vi "Build Installer with API.vi"(8 "error in (no error)":errorcluster, 11 "PostBuildSupport in":refnum<class "PostBuildSupport.lvclass">) -> (0 "error out":errorcluster, 3 "PostBuildSupport out":refnum<class "PostBuildSupport.lvclass">)   [LabVIEW 2016, in "PostBuildSupport.lvclass"]
uses:
  PostBuildSupport.lvclass
  PostBuildSupport.lvclass/PostBuildSupport.ctl
  <vilib>/AppBuilder/IB_Classes/Destination/IB_Destination.lvclass
  <vilib>/AppBuilder/IB_Classes/Source/IB_Source.lvclass
  <vilib>/AppBuilder/IB_Classes/Dest_NI_NIPath/Dest_NI_NIPath.lvclass
  <vilib>/AppBuilder/AB_API/EXE/NI_AB_API_EXE.lvclass
  <vilib>/AppBuilder/IB_Classes/Installer/Installer.lvclass
panel:
  in  "Cancel Button":bool
  out "Progress Bar":u8(slide) caption="The build is complete. You can locate the build at\nC:\\user\\patrick\\git\\PPMS-Monitor-and-Control\\builds\\PPMS Monitor and Control\\Application." scale=0.0..100.0
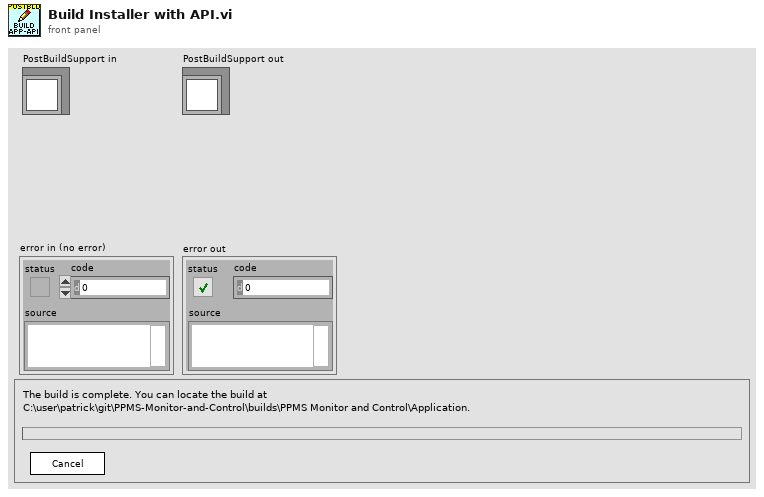
[diagram p1: front panel]
types:
  T1 = enum8{"Enabled", "Disabled", "Disabled and Grayed Out"}
  T2 = typedef "IB_Installer.ctl" = cluster{"Destination":refnum<class "IB_Destination.lvclass">[], "Source":refnum<class "IB_Source.lvclass">[], "buildObject":T3, "defaultDir":string, "platform":string, "author":string, "productName":string, "buildSpecName":string, "hide":bool, "requireLVDevSys":bool, "autoIncrement":bool, "includeError":bool, "readmeID":string, "buildLocation":path, "readmePath":path, "mediaSize":u16, "language":T4, "productVersion":T5, "preview":bool, "programmatic":bool, "progressBarEvents":T6, "userLog_Path":path, "shortcutAddresses":T8[], "EXE_Install Address":string, "EXE_Uninstall Address":string, "additional NIPaths":refnum<class "Dest_NI_NIPath.lvclass">[], "web service itemIDs":string[]}
  T3 = typedef "ItemRef.ctl" = u64
  T4 = typedef "CDK_sTypeDef_Languages.ctl" = u16
  T5 = typedef "CDK_sTypeDef_ProductVersion.ctl" = cluster{"Major":u8, "Minor":u8, "Update":u16}
  T6 = typedef "provcom_ProgressBar_Events.ctl" = cluster{"newJob":refnum<user-event>, "newItem":refnum<user-event>, "errorMsg":T7, "cancel":refnum<user-event>}
  T7 = typedef "mxLvBuildError.ctl" = refnum<user-event>
  T8 = typedef "CDK_sTypeDef_ShortcutAddress.ctl" = cluster{"file":string, "shortcut":string}
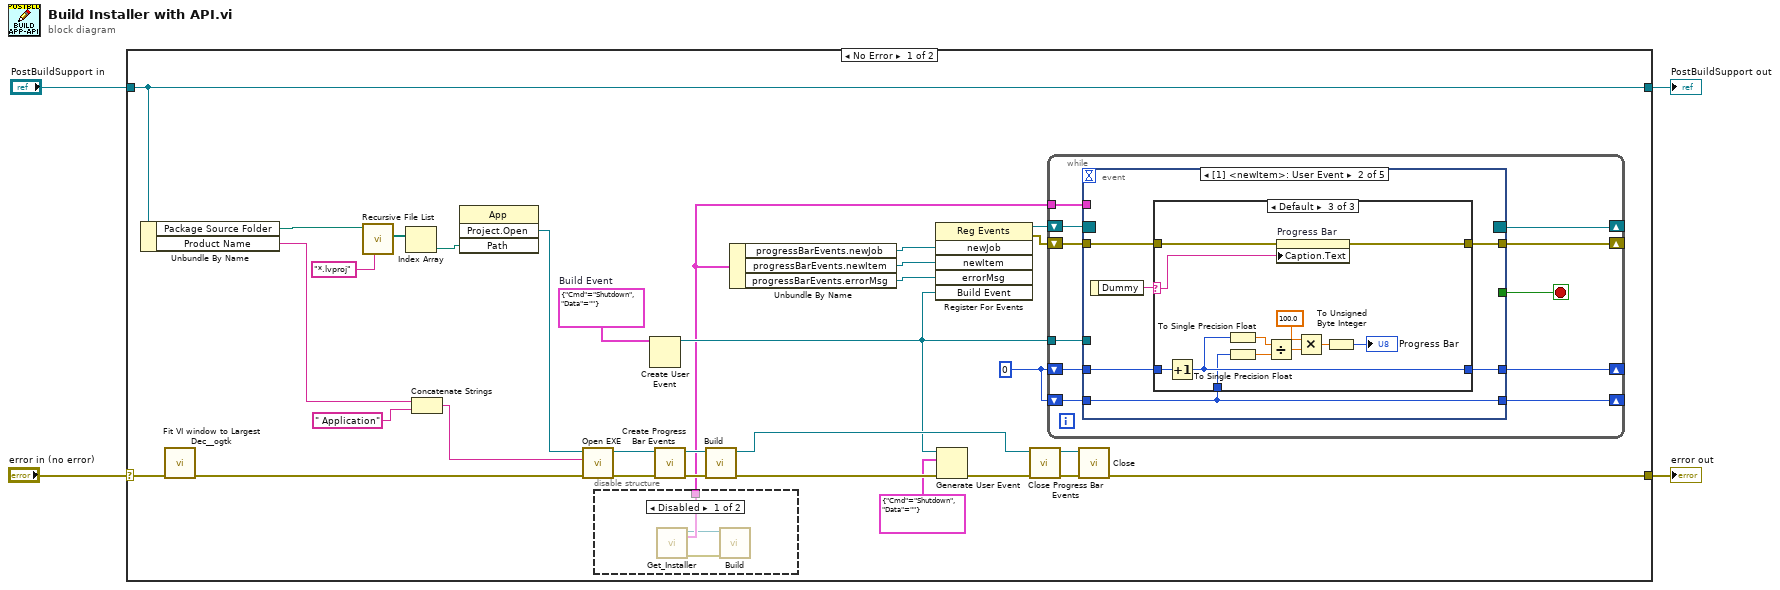
[diagram p0: block diagram]
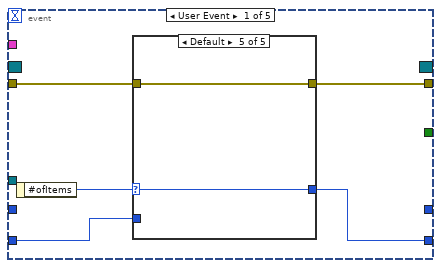
[diagram p3: hidden frame]
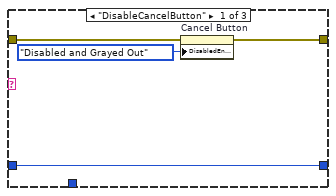
[diagram p8: hidden frame]
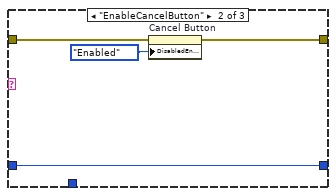
[diagram p9: hidden frame]
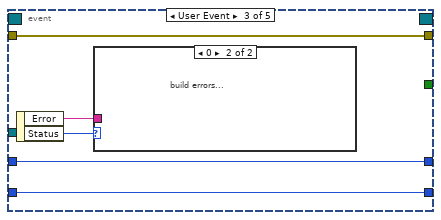
[diagram p10: hidden frame]
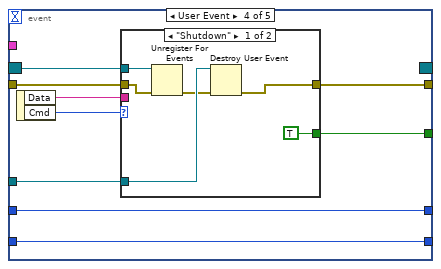
[diagram p12: hidden frame]
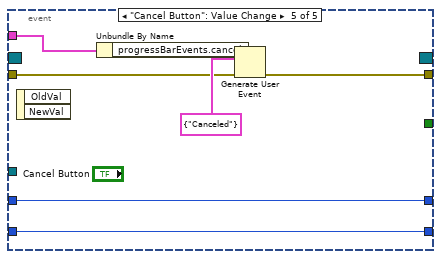
[diagram p14: hidden frame]
diagram:
  n1 = case shown="No Error" "error in (no error)" {
    selector: "error in (no error)" -> [w25 w120]
    tunnel: "PostBuildSupport in" -> [w34 w119]
    tunnel: [w32 w120] -> w2
    tunnel: [w34 w119] -> w1
    frame No Error {
      w13 = cluster{"Cmd":enum16{"Shutdown"}, "Data":string} {"Cmd"=enum."Shutdown", "Data"=""}  # Build Event
      w12 = 0 ("#ofItems")
      n2 = Unbundle By Name(w34) -> ("Package Source Folder"=w28:path, "Product Name"=w29:string)
      n3 = call <userlib>:"Fit VI window to Largest Dec__ogtk.vi"("error in (no error)"=w25) -> ("error out"=w24:errorcluster)  [unwired: 5 in, 1 out]
      n4 = call <vilib>:"Recursive File List.vi"("pattern"="*.lvproj", "Folder Path"=w28) -> ("All Files in Dir"=w35:path[])  [unwired: 5 in, 4 out]
      n5 = Index Array(array=w35) -> (element=w31:path)  [unwired: 1 in]
      n6 = Concatenate Strings(w29, " Application" ("Name of target (My Computer)")) -> (w27:string)
      n7 = invoke class="App" method="Project.Open"("Path"=w31) -> ("Project:Open"=w30:refnum<vi>)  [unwired: 3 in, 3 out]
      n8 = call <vilib>:"Open EXE.vi"("error in (no error)"=w24, "Build specification name"=w27, "Project Refnum"=w30) -> ("error out"=w7:errorcluster, "EXE out"=w5:refnum<class "NI_AB_API_EXE.lvclass">)  [unwired: 7 in]
      n9 = disable-structure shown="Disabled" {
        disable-tunnel: [w38 _] -> w6
        frame Disabled {
          n10 = call <vilib>:"Get_Installer.vi"() -> ("error out"=w37:errorcluster, "data"=w38:T2, "Installer out"=w36:refnum<class "Installer.lvclass">)  [unwired: 9 in]
          n11 = call-dynamic "Build.vi"("error in (no error)"=w37, "Class in"=w36) -> ()  [unwired: 6 in, 4 out]
        }
        frame Enabled {
        }
      }
      n12 = Create User Event(user event datatype=w13) -> (user event=w9:refnum<user-event>)  [unwired: 1 in, 1 out]
      n13 = call-dynamic "Create Progress Bar Events.vi"("error in (no error)"=w7, "NI_AB_API_Build in"=w5) -> ("error out"=w19:errorcluster, "NI_AB_API_Build out"=w23:refnum<class "NI_AB_API_EXE.lvclass">)  [unwired: 7 in, 1 out]
      n14 = call-dynamic "Build.vi"("error in (no error)"=w19, "EXE in"=w23) -> ("error out"=w11:errorcluster, "EXE out"=w22:refnum<class "NI_AB_API_EXE.lvclass">)  [unwired: 6 in, 2 out]
      n15 = Unbundle By Name(w6) -> ("progressBarEvents.newJob"=w18:refnum<user-event>, "progressBarEvents.newItem"=w17:refnum<user-event>, "progressBarEvents.errorMsg"=w16:T7)
      n16 = register-events(w18, w17, w16, w9) -> (reference out=w15:refnum<event-registration>, error out=w14:errorcluster)  [unwired: 2 in]
      n17 = Generate User Event(user event=w9, event data cluster=cluster{"Cmd":enum16{"Shutdown"}, "Data":string} {"Cmd"=enum."Shutdown", "Data"=""} ("event data"), error in=w11) -> (error out=w10:errorcluster)  [unwired: 1 in, 1 out]
      n18 = call-dynamic "Close Progress Bar Events.vi"("error in (no error)"=w10, "NI_AB_API_Build in"=w22) -> ("error out"=w20:errorcluster, "NI_AB_API_Build out"=w21:refnum<class "NI_AB_API_EXE.lvclass">)  [unwired: 8 in]
      n19 = while {
        shift-right: [w49] -> _
        shift-left: w14 -> [w46]
        shift-right: [w48] -> _
        shift-left: w15 -> [w47]
        shift-right: [w44] -> _
        shift-left: w12 -> [w41]
        shift-right: [w43] -> _
        shift-left: w12 -> [w42]
        tunnel: w9 -> [w40]
        tunnel: w6 -> [w39]
        stop <- w45 stop-if-true
        n20 = event shown="[1] <newItem>: User Event" {
          selector: w47 -> [_ _ _ w100 _]
          dyn-events: [_ _ _ _ _] -> w48
          timeout: _ -> [_ _ _ _ _]
          tunnel: [w53 w66 w95 w99 w116] -> w49
          tunnel: w46 -> [w54 w65 w95 w98 w112]
          tunnel: [_ _ _ w102 _] -> w45
          tunnel: [w51 w68 w93 w103 w115] -> w44
          tunnel: [_ w69 w94 w104 w114] -> w43
          tunnel: w42 -> [_ w67 w94 w104 w114]
          tunnel: w41 -> [w50 w68 w93 w103 w115]
          tunnel: w40 -> [_ _ _ w96 _]
          tunnel: w39 -> [_ _ _ _ w113]
          event User Event {
            n21 = event-data() -> ("#ofItems"=w52:i32)  [unwired: 1 in]
            n22 = case shown="Default" w52 {
              selector: w52 -> [w56 w58 w60 _ w64]
              tunnel: w54 -> [w55 w57 w59 w62 w63]
              tunnel: [w55 w57 w59 w62 w63] -> w53
              tunnel: [w56 w58 w60 w61 w64] -> w51
              tunnel: w50 -> [_ _ _ w61 _]
              frame -1 {
                # "Canceled response"
              }
              frame -2 {
              }
              frame -3 {
              }
              frame -4 {
              }
              frame Default {
              }
            }
          }
          event User Event {
            n23 = event-data() -> ("Dummy"=w70:string)  [unwired: 1 in]
            n24 = case shown="Default" w70 {
              selector: w70 -> [_ _ w81]
              tunnel: w67 -> [w73 w77 w88]
              tunnel: [w73 w77 w87] -> w69
              tunnel: w68 -> [_ _ w86]
              tunnel: [w71 w75 w79] -> w66
              tunnel: w65 -> [w72 w76 w80]
              frame "DisableCancelButton" {
                n25 = property on="Cancel Button" class="Bool"(error in=w72, "DisabledEnum"=T1."Disabled and Grayed Out" ("Disabled")) -> (error out=w71:errorcluster)  [unwired: 1 in, 1 out]
              }
              frame "EnableCancelButton" {
                n26 = property on="Cancel Button" class="Bool"(error in=w76, "DisabledEnum"=T1."Enabled" ("Disabled")) -> (error out=w75:errorcluster)  [unwired: 1 in, 1 out]
              }
              frame Default {
                n27 = Increment(x=w88) -> (x+1=w87:i32)
                n28 = To Single Precision Float(number=w87) -> (single precision float=w84:sgl)
                n29 = To Single Precision Float(number=w86) -> (single precision float=w83:sgl)
                n30 = Divide(x=w84, y=w83) -> (x/y=w85:sgl)
                n31 = property on="Progress Bar" class="Slide (strict)"(error in=w80, "Caption.Text"=w81) -> (error out=w79:errorcluster)  [unwired: 1 in, 1 out]
                n32 = Multiply(x=sgl 100.0, y=w85) -> (x*y=w90:sgl)
                n33 = To Unsigned Byte Integer(number=w90) -> (unsigned 8bit integer=→"Progress Bar":u8)
              }
            }
          }
          event User Event {
            n34 = event-data() -> ("Error"=w91:string, "Status"=w92:i32)  [unwired: 1 in]
            n35 = case shown="0" w92 {
              tunnel: w91 -> [_ _]
              frame Default {
              }
              frame 0 {
                # "build errors..."
              }
            }
          }
          event User Event {
            n36 = event-data() -> ("Data"=w97:string, "Cmd"=w101:enum16{"Shutdown"})  [unwired: 1 in]
            n37 = case shown="\"Shutdown\"" w101 {
              tunnel: [TRUE _] -> w102
              tunnel: w100 -> [w109 _]
              tunnel: [w105 w111] -> w99
              tunnel: w98 -> [w108 w111]
              tunnel: w97 -> [_ _]
              tunnel: w96 -> [w107 _]
              frame "Shutdown" {
                n38 = Unregister For Events(event registration refnum=w109, error in=w108) -> (error out=w106:errorcluster)
                n39 = Destroy User Event(user event=w107, error in=w106) -> (error out=w105:errorcluster)
              }
              frame Default {
              }
            }
          }
          event "Cancel Button": Value Change {
            n40 = event-data() -> ()  [unwired: 1 in, 2 out]
            n41 = Unbundle By Name(w113) -> ("progressBarEvents.cancel"=w117:refnum<user-event>)
            n42 = Generate User Event(user event=w117, event data cluster=cluster{"Dummy":string} {"Dummy"="Canceled"} ("event data"), error in=w112) -> (error out=w116:errorcluster)  [unwired: 1 in, 1 out]
          }
        }
      }
      n43 = call-dynamic "Close.vi"("error in (no error)"=w20, "EXE in"=w21) -> ("error out"=w32:errorcluster)  [unwired: 9 in]
    }
    frame Error {
    }
  }
  "error out" <- w2
  "PostBuildSupport out" <- w1
